vi "Resolution.vi"(8 "error in (no error)":errorcluster, 9 "Resolution":T2, 11 "Reference in":T1={"Device"="GPIB0::4::INSTR", "Function"="", "delay"=20, "Resolution"=0}) -> (0 "error out":errorcluster, 3 "Reference out":T1={"Device"="GPIB0::4::INSTR", "Function"="", "delay"=20, "Resolution"=0}, 4 "question out":string)   [LabVIEW 2021, in "Rigol DM3052.lvlib"]
uses:
  Rigol DM3052.lvlib
  Resolution.ctl
  Reference.ctl
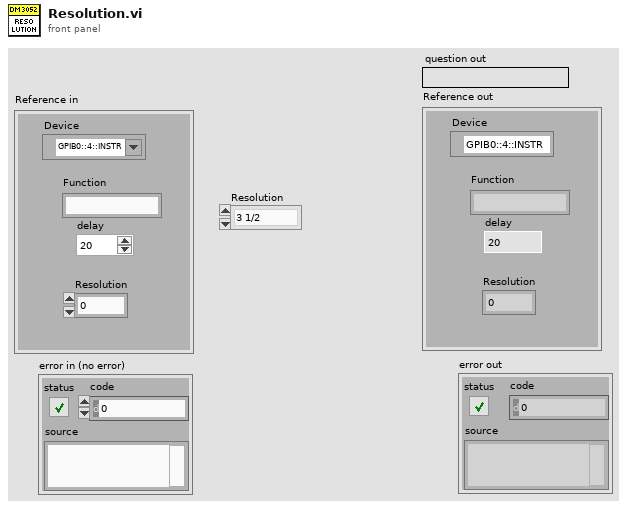
[diagram p1: front panel]
types:
  T1 = typedef "Rigol DM3052.lvlib/Reference.ctl" = cluster{"Device":refnum<visa-resource-name>, "Function":string, "delay":u32, "Resolution":i8}
  T2 = typedef "Rigol DM3052.lvlib/Resolution.ctl" = enum16{"3 1/2", "4 1/2", "5 1/2"}
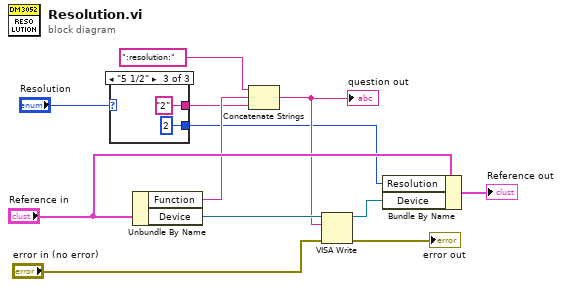
[diagram p0: block diagram]
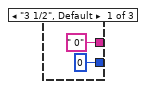
[diagram p2: hidden frame]
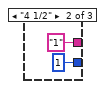
[diagram p3: hidden frame]
diagram:
  n1 = case shown="\"5 1/2\"" "Resolution" {
    tunnel: [" 0" "1" "2"] -> w2
    tunnel: [i8 0 ("Resolution") i8 1 ("Resolution") i8 2 ("Resolution")] -> w1
    frame "3 1/2", Default {
    }
    frame "4 1/2" {
    }
    frame "5 1/2" {
    }
  }
  n2 = Unbundle By Name("Reference in") -> ("Function"=w3:string, "Device"=w11:refnum<visa-resource-name>)
  n3 = Concatenate Strings(":resolution:", w3, w2) -> (w8:string)
  "question out" <- w8
  n4 = VISA Write(VISA resource name=w11, write buffer=w8, error in (no error)="error in (no error)") -> (VISA resource name out=w6:refnum<visa-resource-name>, error out=→"error out":errorcluster)  [unwired: 1 out]
  n5 = Bundle By Name(cluster="Reference in", "Resolution"=w1, "Device"=w6) -> (→"Reference out":T1)
